vi "DiffVI.vi"(8 "error in (no error)":errorcluster) -> (0 "error out":errorcluster)   [LabVIEW 2020, in "CICD.lvlib"]
doc: "Use GCLI to call the DiffVI method.\nThis method accepts the following input parameters:\n- PathToOldVI\n-PathToNewVI\n-OutputDir"
uses:
  CICD.lvlib
  <vilib>/Wiresmith Technology/G CLI/Argument Parser/Option Class/Option Configuration.ctl
  <vilib>/Wiresmith Technology/G CLI/Argument Parser/Option Class/Argument Type.ctl
  <vilib>/Wiresmith Technology/G CLI/CLI Class/CLI.lvclass
  <vilib>/Wiresmith Technology/G CLI/Argument Parser/Option Set Class/Option Set.lvclass
  <vilib>/Wiresmith Technology/G CLI/Argument Parser/Option Class/Option.lvclass
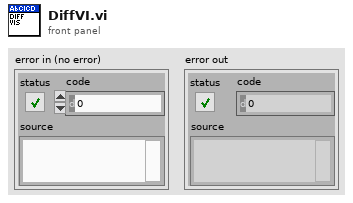
[diagram p1: front panel]
types:
  T1 = typedef "Option Parser.lvlib/Option.lvclass/Option Configuration.ctl" = cluster{"Option Type":T2, "Option Labels":string[], "Key":string, "Description":string, "Required":bool, "Default Value":string}
  T2 = typedef "Option Parser.lvlib/Option.lvclass/Argument Type.ctl" = enum16{"flag", "value"}
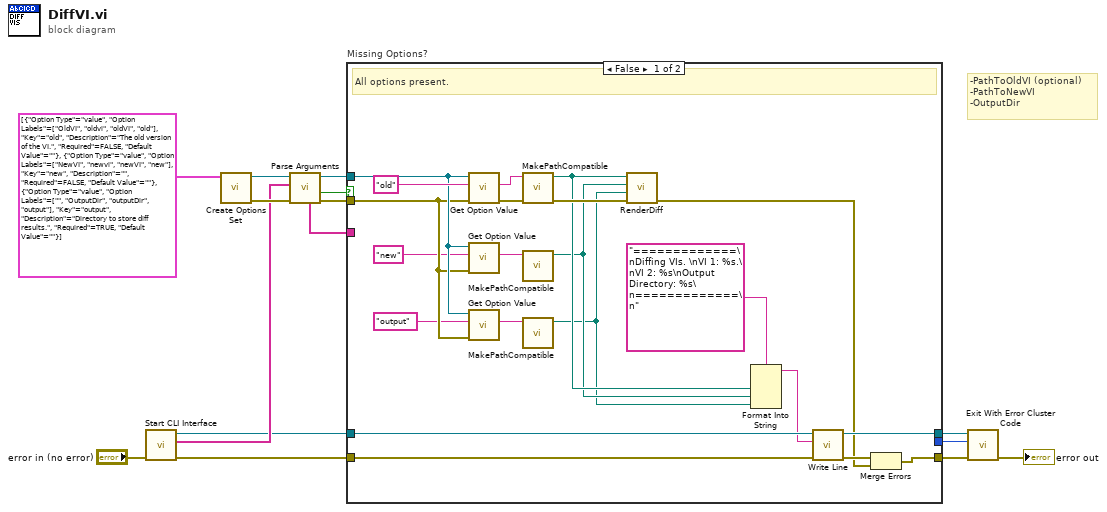
[diagram p0: block diagram]
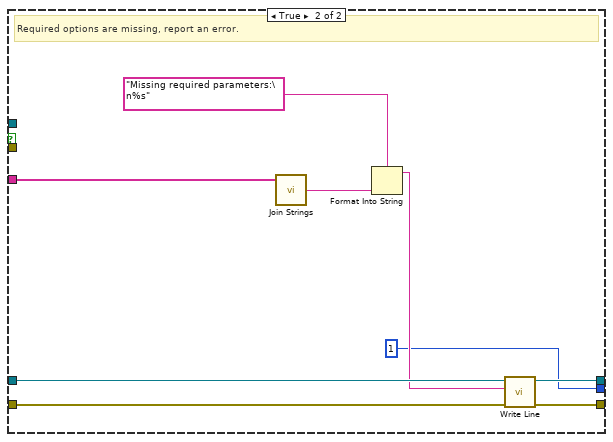
[diagram p2: hidden frame]
diagram:
  # "-PathToOldVI (optional)\n-PathToNewVI\n-OutputDir"
  n1 = call <vilib>:"Start CLI Interface.vi"("error in (no error)"="error in (no error)") -> ("error out"=w7:errorcluster, "Custom Parameters"=w11:string[], "CLI out"=w6:refnum<class "CLI.lvclass">)  [unwired: 7 in, 1 out]
  n2 = call <vilib>:"Create Options Set.vi"("Options"=T1[] [{"Option Type"=enum."value", "Option Labels"=["OldVI", "oldvi", "oldVI", "old"], "Key"="old", "Description"="The old version of the VI.", "Required"=FALSE, "Default Value"=""}, {"Option Type"=enum."value", "Option Labels"=["NewVI", "newvi", "newVI", "new"], "Key"="new", "Description"="", "Required"=FALSE, "Default Value"=""}, {"Option Type"=enum."value", "Option Labels"=["", "OutputDir", "outputDir", "output"], "Key"="output", "Description"="Directory to store diff results.", "Required"=TRUE, "Default Value"=""}]) -> ("error out"=w13:errorcluster, "Option Set out"=w14:refnum<class "Option Set.lvclass">)  [unwired: 9 in]
  n3 = call <vilib>:"Parse Arguments.vi"("error in (no error)"=w13, "Arguments"=w11, "Option Set in"=w14) -> ("error out"=w9:errorcluster, "Missing Options"=w10:bool, "Option Set out"=w1:refnum<class "Option Set.lvclass">, "Missing Option Keys"=w8:string[])  [unwired: 5 in]
  n4 = case "Missing Options?" shown="False" w10 {
    tunnel: w9 -> [w27 _]
    tunnel: w8 -> [_ w42]
    tunnel: w7 -> [w35 w41]
    tunnel: w6 -> [w32 w40]
    tunnel: [w30 w38] -> w5
    tunnel: [w31 w37] -> w3
    tunnel: [_ 1 ("No Error Code (0)")] -> w2
    tunnel: w1 -> [w28 _]
    frame False {
      # "All options present."
      n5 = call <vilib>:"Get Option Value.vi"("error in (no error)"=w27, "Option Key"="old", "Option Set in"=w28) -> ("error out"=w25:errorcluster, "Value"=w21:string)  [unwired: 5 in, 2 out]
      n6 = call <vilib>:"Get Option Value.vi"("error in (no error)"=w27, "Option Key"="new", "Option Set in"=w28) -> ("Value"=w20:string)  [unwired: 5 in, 3 out]
      n7 = call <vilib>:"Get Option Value.vi"("error in (no error)"=w27, "Option Key"="output", "Option Set in"=w28) -> ("Value"=w19:string)  [unwired: 5 in, 3 out]
      n8 = call "MakePathCompatible.vi"("path string"=w21) -> ("path"=w18:path)  [unwired: 10 in]
      n9 = call "MakePathCompatible.vi"("path string"=w20) -> ("path"=w17:path)  [unwired: 10 in]
      n10 = call "MakePathCompatible.vi"("path string"=w19) -> ("path"=w16:path)  [unwired: 10 in]
      n11 = call "RenderDiff.vi"("error in (no error)"=w25, "-OutputDir"=w16, "-PathToNewVI"=w17, "-PathToOldVI"=w18) -> ("error out"=w23:errorcluster)  [unwired: 7 in]
      n12 = Format Into String(format string="=============\nDiffing VIs. \nVI 1: %s.\nVI 2: %s\nOutput Directory: %s\n=============\n", w18, w17, w16) -> (resulting string=w29:string)  [unwired: 2 in, 1 out]
      n13 = call <vilib>:"Write Line.vi"("error in (no error)"=w35, "Text to Write"=w29, "CLI in"=w32) -> ("error out"=w33:errorcluster, "CLI out"=w31:refnum<class "CLI.lvclass">)  [unwired: 7 in]
      n14 = Merge Errors(w33, w23) -> (w30:errorcluster)
    }
    frame True {
      # "Required options are missing, report an error."
      n15 = call <vilib>:"Join Strings.vi"("Strings In"=w42) -> ("String"=w43:string)  [unwired: 2 in]
      n16 = Format Into String(format string="Missing required parameters:\n%s" ("Text to Write"), w43) -> (resulting string=w39:string)  [unwired: 2 in, 1 out]
      n17 = call <vilib>:"Write Line.vi"("error in (no error)"=w41, "Text to Write"=w39, "CLI in"=w40) -> ("error out"=w38:errorcluster, "CLI out"=w37:refnum<class "CLI.lvclass">)  [unwired: 7 in]
    }
  }
  n18 = call <vilib>:"Exit With Error Cluster Code.vi"("error in (no error)"=w5, "No Error Code (0)"=w2, "CLI in"=w3) -> ("error out"=→"error out":errorcluster)  [unwired: 8 in]
